vi "VCI_SetReference2.vi"(6 "Data":variant, 7 "RefType":T1 items=["MODE"=0, "FILTER"=1, "ACR"=2, "AMR"=6, "kCANBAUD"=10, "TIMING0"=11, "TIMING1"=12, "CANRX_EN"=13, "UARTBAUD"=14, "RefNormal"=15, "BaudType"=16], 8 "error in (no error)":errorcluster caption="错误输入（无错误）", 9 "CANIndex":u32, 10 "DevIndex":u32, 11 "DevType":T2=2 items=["USB-CAN"=2, "USB-CAN2"=3]) -> (0 "error out":errorcluster caption="错误输出", 3 "Return Val":T3=1 items=["OK"=1, "ERROR1"=0, "ERROR2"=-1])   [LabVIEW 2018, in "ControlCan.lvlib"]
uses:
  ControlCan.lvlib
  Return Val.ctl
  DevType.ctl
  RefType.ctl
  RefNormal.ctl
  Mode.ctl
  Fliter.ctl
  kBaudRate.ctl
  BaudType.ctl
  SJW.ctl
  BRP.ctl
  SAM.ctl
  PHSEG2_SEL.ctl
  PRSEG.ctl
  PHSEG1.ctl
  PHSEG2.ctl
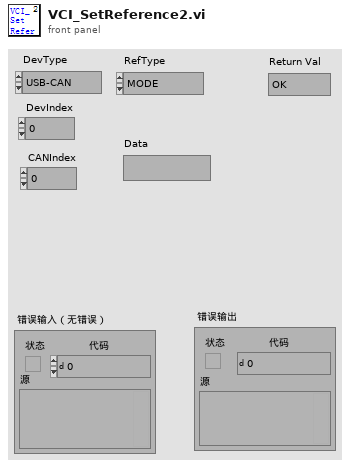
[diagram p1: front panel]
types:
  T1 = typedef "ControlCAN.lvlib/RefType.ctl" = u32
  T2 = typedef "ControlCAN.lvlib/DevType.ctl" = u32
  T3 = typedef "ControlCAN.lvlib/Return Val.ctl" = i32
  T4 = typedef "ControlCAN.lvlib/RefNormal.ctl" = cluster{"Mode":T5, "Fliter":T6, "AccCode":u32, "AccMask":u32, "kBaudRate":T7, "Timing0":u8, "Timing1":u8, "CANRX_EN":u8, "UARTBAUD":u8}
  T5 = typedef "ControlCAN.lvlib/Mode.ctl" = u8
  T6 = typedef "ControlCAN.lvlib/Fliter.ctl" = u8
  T7 = typedef "ControlCAN.lvlib/kBaudRate.ctl" = u8
  T8 = typedef "ControlCAN.lvlib/BaudType.ctl" = cluster{"Baud":u32, "SJW":T9, "BRP":T10, "SAM":T11, "PHSEG2_SEL":T12, "PRSEG":T13, "PHSEG1":T14, "PHSEG2":T15}
  T9 = typedef "ControlCAN.lvlib/SJW.ctl" = u8
  T10 = typedef "ControlCAN.lvlib/BRP.ctl" = u8
  T11 = typedef "ControlCAN.lvlib/SAM.ctl" = u8
  T12 = typedef "ControlCAN.lvlib/PHSEG2_SEL.ctl" = u8
  T13 = typedef "ControlCAN.lvlib/PRSEG.ctl" = u8
  T14 = typedef "ControlCAN.lvlib/PHSEG1.ctl" = u8
  T15 = typedef "ControlCAN.lvlib/PHSEG2.ctl" = u8
  T16 = typedef "ControlCAN.lvlib/RefNormal_1.ctl" = cluster{"Mode":T5, "Fliter":T6, "AccCode 0":u8, "AccCode 1":u8, "AccCode 2":u8, "AccCode 3":u8, "AccMask 0":u8, "AccMask 1":u8, "AccMask 2":u8, "AccMask 3":u8, "kBaudRate":T7, "Timing0":u8, "Timing1":u8, "CANRX_EN":u8, "UARTBAUD":u8}
  T17 = typedef "ControlCAN.lvlib/BaudType_1.ctl" = cluster{"Baud 0":u8, "Baud 1":u8, "Baud 2":u8, "Baud 3":u8, "SJW":T9, "BRP":T10, "SAM":T11, "PHSEG2_SEL":T12, "PRSEG":T13, "PHSEG1":T14, "PHSEG2":T15}
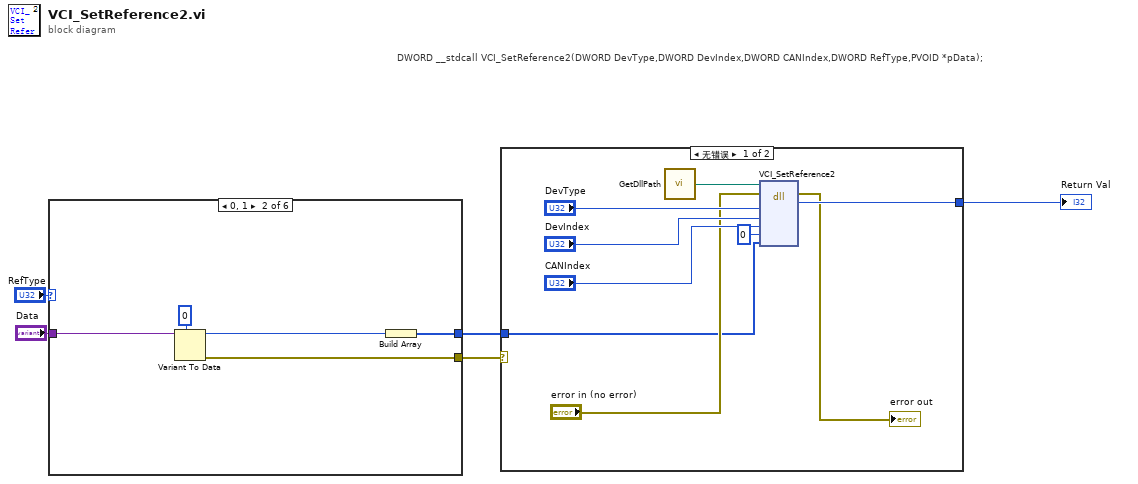
[diagram p0: block diagram]
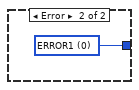
[diagram p2: hidden frame]
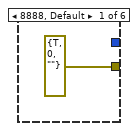
[diagram p3: hidden frame]
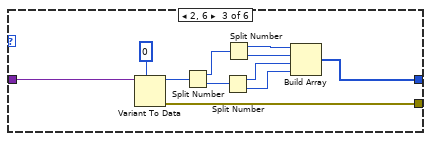
[diagram p4: hidden frame]
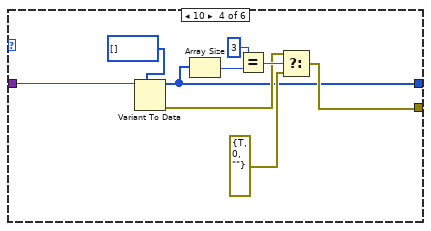
[diagram p5: hidden frame]
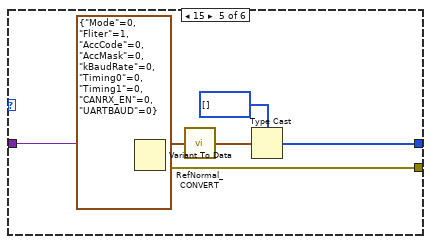
[diagram p6: hidden frame]
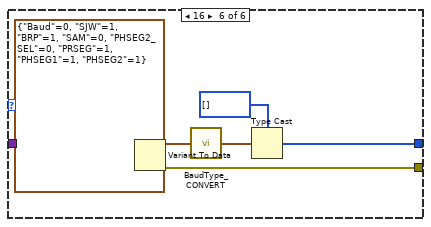
[diagram p7: hidden frame]
diagram:
  # "DWORD __stdcall VCI_SetReference2(DWORD DevType,DWORD DevIndex,DWORD CANIndex,DWORD RefType,PVOID *pData);"
  n1 = case shown="0, 1" "RefType" {
    tunnel: "Data" -> [_ w11 w22 w31 w38 w45]
    tunnel: [errorcluster {"status"=TRUE, "code"=0, "source"=""} ("error constant") w10 w21 w24 w37 w44] -> w2
    tunnel: [_ w8 w12 w23 w32 w42] -> w1
    frame 8888, Default {
    }
    frame 0, 1 {
      n2 = Variant To Data(type=u8 0, Variant=w11) -> (data=w9:u8, error out=w10:errorcluster)  [unwired: 1 in]
      n3 = Build Array(w9) -> (w8:u8[])
    }
    frame 2, 6 {
      n4 = Variant To Data(type=u32 0, Variant=w22) -> (data=w19:u32, error out=w21:errorcluster)  [unwired: 1 in]
      n5 = Split Number(x=w19) -> (hi(x)=w18:u16, lo(x)=w17:u16)
      n6 = Split Number(x=w17) -> (hi(x)=w14:u8, lo(x)=w13:u8)
      n7 = Split Number(x=w18) -> (hi(x)=w16:u8, lo(x)=w15:u8)
      n8 = Build Array(w16, w15, w14, w13) -> (w12:u8[])
    }
    frame 10 {
      n9 = Variant To Data(type=u8[] [] ("添加的数组"), Variant=w31) -> (data=w23:u8[], error out=w26:errorcluster)  [unwired: 1 in]
      n10 = Array Size(array=w23) -> (size(s)=w29:i32)
      n11 = Equal?(x=3, y=w29) -> (x = y?=w27:bool)
      n12 = Select(t=w26, s=w27, f=errorcluster {"status"=TRUE, "code"=0, "source"=""} ("error constant")) -> (s? t:f=w24:errorcluster)
    }
    frame 15 {
      n13 = Variant To Data(type=T4 {"Mode"=0, "Fliter"=1, "AccCode"=0, "AccMask"=0, "kBaudRate"=0, "Timing0"=0, "Timing1"=0, "CANRX_EN"=0, "UARTBAUD"=0} ("RefNormal"), Variant=w38) -> (data=w35:T4, error out=w37:errorcluster)  [unwired: 1 in]
      n14 = call "RefNormal_CONVERT.vi"("RefNormal"=w35) -> ("RefNormal_1"=w34:T16)
      n15 = Type Cast(type=u8[] [] ("添加的数组"), x=w34) -> (*(type *) &x=w32:u8[])
    }
    frame 16 {
      n16 = Variant To Data(type=T8 {"Baud"=0, "SJW"=1, "BRP"=1, "SAM"=0, "PHSEG2_SEL"=0, "PRSEG"=1, "PHSEG1"=1, "PHSEG2"=1} ("BaudType"), Variant=w45) -> (data=w40:T8, error out=w44:errorcluster)  [unwired: 1 in]
      n17 = call "BaudType_CONVERT.vi"("BaudType"=w40) -> ("BaudType_1"=w39:T17)
      n18 = Type Cast(type=u8[] [] ("添加的数组"), x=w39) -> (*(type *) &x=w42:u8[])
    }
  }
  n19 = case shown="无错误" w2 {
    tunnel: [w53 w55] -> w5
    tunnel: w1 -> [w48 _]
    frame No Error {
      n20 = call "GetDllPath.vi"() -> ("DllPath"=w46:path)  [unwired: 1 in]
      n21 = dll-call lib="?" fn="VCI_SetReference2"(path in=w46, error in="error in (no error)", "DevType"="DevType", "DevIndex"="DevIndex", "CANIndex"="CANIndex", "RefType"=u32 0, "pData"=w48) -> (error out=→"error out":errorcluster, "ReturnVal"=w53:i32)  [unwired: 6 in, 1 out]
    }
    frame Error {
      w55 = T3 0 items=["OK"=1, "ERROR1"=0, "ERROR2"=-1] ("Return Val")
    }
  }
  "Return Val" <- w5
